vi "2ch_rawcdc_protocol.vi"() -> ()   [LabVIEW 2020]
doc: "This example performs writes and reads on a serial port, as directed by the user. You can press the Write and Read buttons, and change the Read Count, while the example is running.\n\nThe parameters set for the serial port must match the parameters of the connected instrument or device. In this example, the Read Count parameter specifies the number of bytes that the serial port reads. If there were more bytes at the port than the specified number, those bytes would not be read. If there were less bytes at the port than the specified number, you would receive a timeout error.\n\nThis example expands upon the flow control options for XON and XOFF, allowing the user to choose those control characters. Also, the user can enable or disable a termination character. Some devices require a termination character in order to identify the end of command strings. Some devices send a termination character to signify the end of data to be read. This example shows how you can end the Read operation once a termination character is detected in the buffer and/or append a termination character at the end of the Write data."
uses:
  <vilib>/Instr/_visa.llb/VISA Configure Serial Port (Instr).vi
panel:
  out "Waveform Chart":dbl[][](graph)
  in  "Command List":string="stop\nencode 0\nslist 0 0\nslist 1 1\nsrate 6000\nps 2\ndec 1\ndeca 3\nnop\n\n\n"
  in  "Stop":bool
  in  "2108 CDC Virtual COM":refnum<visa-resource-name>="COM11"
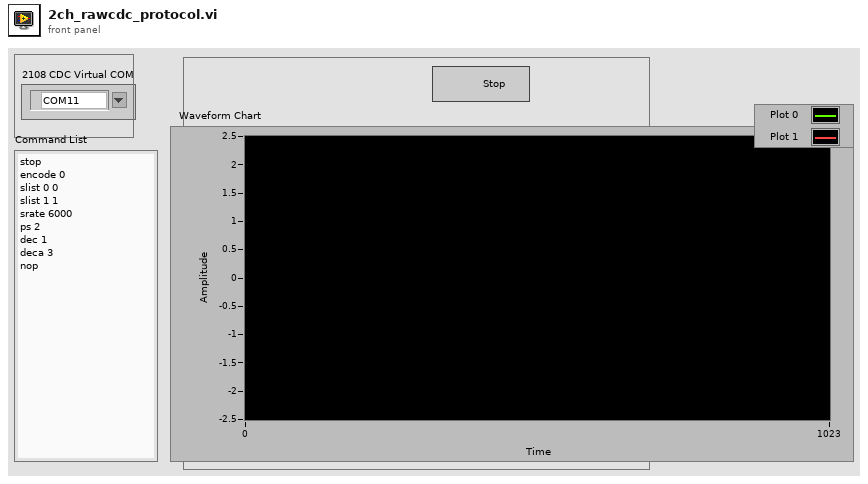
[diagram p1: front panel]
types:
  T1 = enum16{"big-endian, network order", "native, host order", "little-endian"}
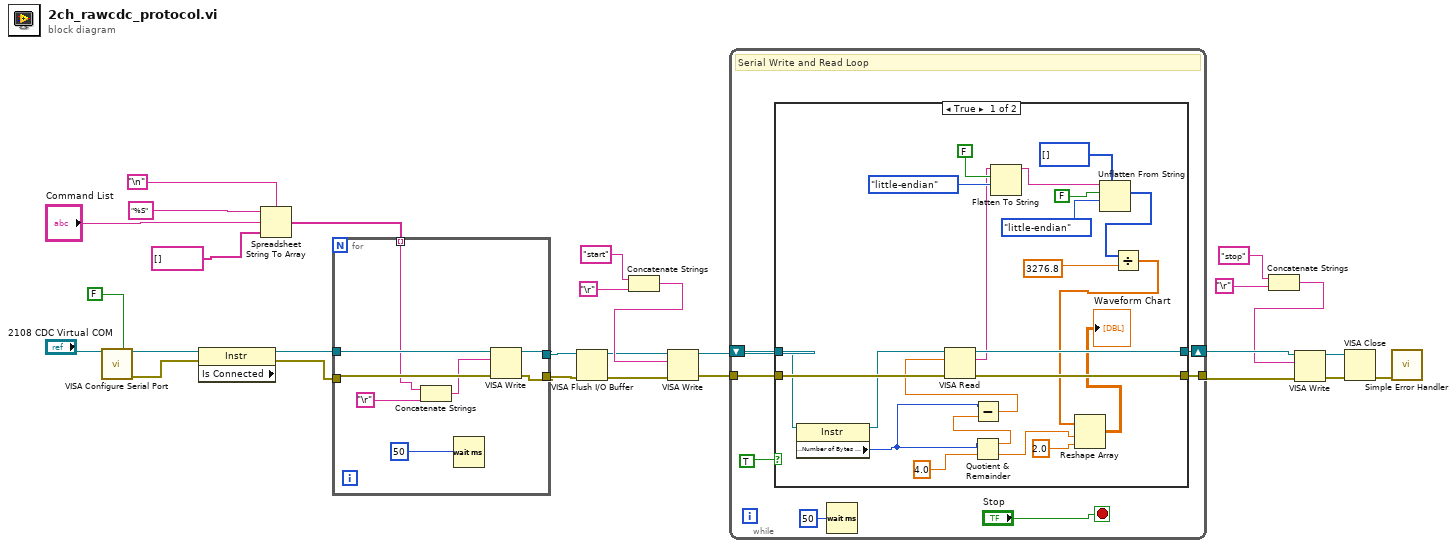
[diagram p0: block diagram]
diagram:
  n1 = call-poly "VISA Configure Serial Port"("VISA resource name"="2108 CDC Virtual COM", "Enable Termination\nChar (T)"=FALSE) -> ("VISA resource name out"=w26:refnum<visa-resource-name>, "error out"=w28:errorcluster)  [unwired: 8 in, 4 out]
  n2 = property class="Instr" props=["Is Connected"](reference=w26, error in=w28) -> (reference out=w2:refnum<visa-resource-name>, error out=w1:errorcluster)  [unwired: 1 out]
  n3 = Spreadsheet String To Array(delimiter (Tab)="\n", format string="%S", spreadsheet string="Command List", array type (2D Dbl)=string[] []) -> (array=w22:string[])
  n4 = for {
    tunnel: w22 -> [w33] mode=indexing
    tunnel: w2 -> [w36]
    tunnel: w1 -> [w35]
    tunnel: [w30] -> w6
    tunnel: [w29] -> w4
    n5 = Concatenate Strings(w33, "\r") -> (w31:string)
    n6 = Wait (ms)(milliseconds to wait=u32 50) -> ()  [unwired: 1 out]
    n7 = VISA Write(VISA resource name=w36, write buffer=w31, error in (no error)=w35) -> (VISA resource name out=w30:refnum<visa-resource-name>, error out=w29:errorcluster)  [unwired: 1 out]
  }
  n8 = VISA Flush I/O Buffer(VISA resource name=w6, error in (no error)=w4) -> (VISA resource name out=w5:refnum<visa-resource-name>, error out=w3:errorcluster)  [unwired: 1 in]
  n9 = Concatenate Strings("start", "\r") -> (w10:string)
  n10 = VISA Write(VISA resource name=w5, write buffer=w10, error in (no error)=w3) -> (VISA resource name out=w9:refnum<visa-resource-name>, error out=w8:errorcluster)  [unwired: 1 out]
  n11 = while {
    shift-right: [w43] -> w19
    shift-left: w9 -> [w39]
    tunnel: w8 -> [w38]
    tunnel: [w41] -> w16
    stop <- "Stop" stop-if-true
    # "Serial Write and Read Loop"
    n12 = case shown="True" TRUE {
      tunnel: [w64 w67] -> w43
      tunnel: w39 -> [w62 w67]
      tunnel: w38 -> [w65 w66]
      tunnel: [w57 w66] -> w41
      frame True {
        n13 = property class="Instr"(reference=w62) -> (reference out=w56:refnum<visa-resource-name>, "Serial Settings:Number of Bytes at Serial Port"=w61:u32)  [unwired: 1 in, 1 out]
        n14 = Quotient & Remainder(x=w61, y=4.0) -> (x-y*floor(x/y)=w59:dbl, floor(x/y)=w45:dbl)
        n15 = Subtract(x=w61, y=w59) -> (x-y=w58:dbl)
        n16 = VISA Read(VISA resource name=w56, byte count=w58, error in (no error)=w65) -> (VISA resource name out=w64:refnum<visa-resource-name>, read buffer=w50:string, error out=w57:errorcluster)  [unwired: 1 out]
        n17 = Flatten To String(anything=w50, prepend array or string size? (T)=FALSE, byte order (0:big-endian, network order)=T1."little-endian") -> (data string=w51:string)  [unwired: 1 in, 2 out]
        n18 = Unflatten From String(type=i16[] [], binary string=w51, data includes array or string size? (T)=FALSE, byte order (0:big-endian, network order)=T1."little-endian") -> (value=w49:i16[])  [unwired: 1 in, 2 out]
        n19 = Divide(x=w49, y=3276.8) -> (x/y=w47:dbl[])
        n20 = Reshape Array(w47, w45, 2.0) -> (→"Waveform Chart":dbl[][])
      }
      frame False {
      }
    }
    n21 = Wait (ms)(milliseconds to wait=u32 50) -> ()  [unwired: 1 out]
  }
  n22 = Concatenate Strings("stop", "\r") -> (w13:string)
  n23 = VISA Write(VISA resource name=w19, write buffer=w13, error in (no error)=w16) -> (VISA resource name out=w18:refnum<visa-resource-name>, error out=w17:errorcluster)  [unwired: 1 out]
  n24 = VISA Close(VISA resource name=w18, error in (no error)=w17) -> (error out=w27:errorcluster)
  n25 = call <vilib>:"Simple Error Handler.vi"("error in (no error)"=w27) -> ()  [unwired: 1 in, 8 out]
